vi "Take Single Sample.vi"(8 "error in (no error)":errorcluster, 11 "Refnum in":refnum<k21>) -> (0 "error out":errorcluster, 1 "Mean Voltage Detected":dbl format="%0.2f", 3 "Refnum out":refnum<k21>)   [LabVIEW 2021]
uses:
  <vilib>/DAQmx/read.llb/DAQmx Read (Analog DBL 1Chan 1Samp).vi
  <vilib>/DAQmx/miscellaneous.llb/DAQmx Fill In Error Info.vi
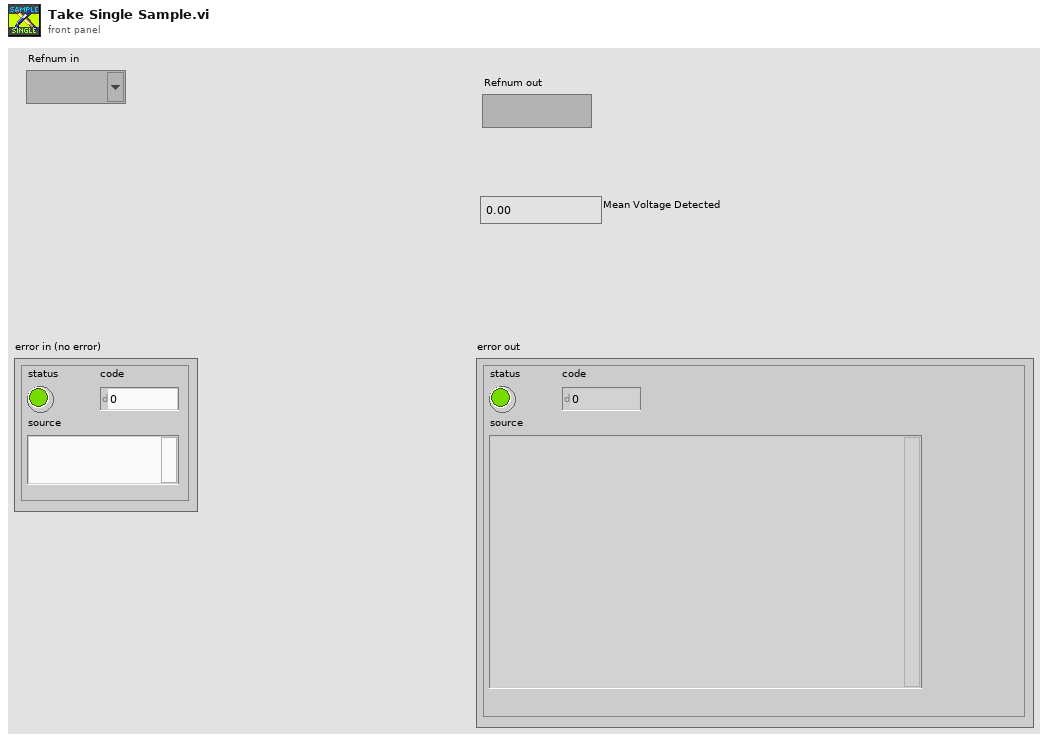
[diagram p1: front panel]
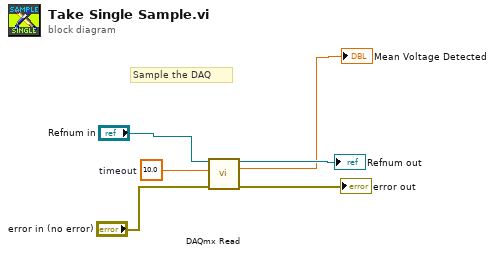
[diagram p0: block diagram]
diagram:
  w4 = 10.0  # timeout
  # "Sample the DAQ"
  n1 = call-poly <vilib>:"DAQmx Read.vi"("task/channels in"="Refnum in", "timeout"=w4, "error in"="error in (no error)") -> ("task out"=→"Refnum out":refnum<k21>, "data"=→"Mean Voltage Detected":dbl, "error out"=→"error out":errorcluster)  [unwired: 10 in]
